vi "DAQ_ReadMeasurements.vi"(0 "task/channels in":refnum<k21>, 7 "error in":errorcluster) -> (20 "task out":refnum<k21>, 21 "Measurements":T1, 22 "Raw Temperature Voltage (V)":dbl, 23 "Raw Current Voltage (V)":dbl, 24 "Raw Torque Voltage (V)":dbl, 25 "Raw Vibration Voltage (V)":dbl, 26 "Raw RPM Voltage (V)":dbl, 27 "error out":errorcluster)   [LabVIEW 2026]
uses:
  MotorMeasurements.ctl
  <vilib>/DAQmx/read.llb/DAQmx Read (Analog 1D DBL NChan 1Samp).vi
  <vilib>/DAQmx/miscellaneous.llb/DAQmx Fill In Error Info.vi
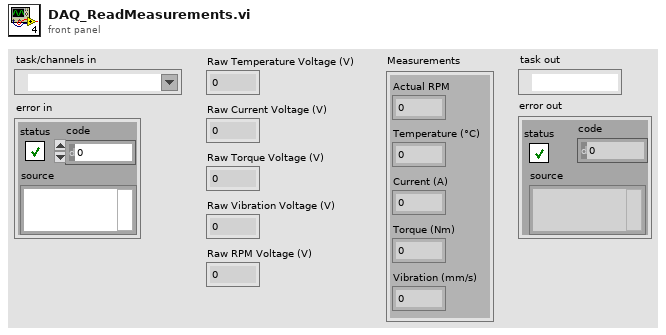
[diagram p1: front panel]
types:
  T1 = typedef "MotorMeasurements.ctl" = cluster{"Temperature (°C)":dbl, "Current (A)":dbl, "Torque (Nm)":dbl, "Vibration (mm/s)":dbl, "Actual RPM":dbl}
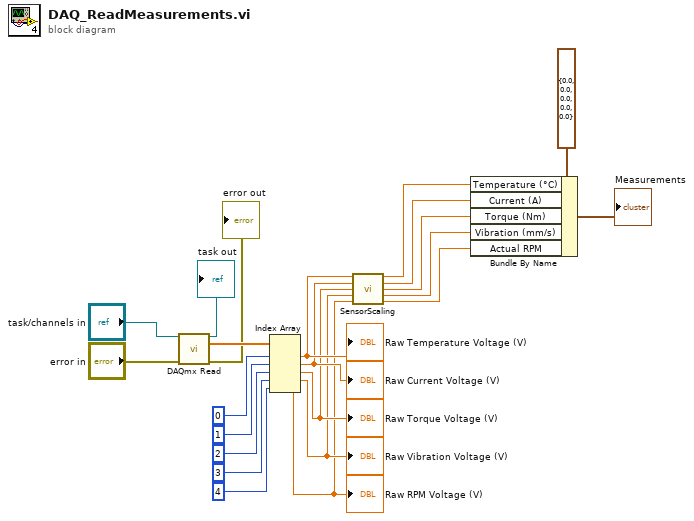
[diagram p0: block diagram]
diagram:
  n1 = call-poly <vilib>:"DAQmx Read.vi"("task/channels in"="task/channels in", "error in"="error in") -> ("task out"=→"task out":refnum<k21>, "data"=w16:dbl[], "error out"=→"error out":errorcluster)  [unwired: 11 in]
  n2 = Index Array(array=w16, index #1=0 ("index"), index #2=1 ("index"), index #3=2 ("index"), index #4=3 ("index"), index #5=4 ("index")) -> (element #1=w15:dbl, element #2=w14:dbl, element #3=w4:dbl, element #4=w3:dbl, element #5=w2:dbl)
  "Raw Temperature Voltage (V)" <- w15
  "Raw Current Voltage (V)" <- w14
  "Raw Torque Voltage (V)" <- w4
  "Raw Vibration Voltage (V)" <- w3
  "Raw RPM Voltage (V)" <- w2
  n3 = call "SensorScaling.vi"("Temperature Voltage (V)"=w15, "Current Voltage (V)"=w14, "Torque Voltage (V)"=w4, "Vibration Voltage (V)"=w3, "RPM Voltage (V)"=w2) -> ("Temperature (°C)"=w9:dbl, "Current (A)"=w8:dbl, "Torque (Nm)"=w6:dbl, "Vibration (mm/s)"=w5:dbl, "Actual RPM"=w1:dbl)  [unwired: 6 in]
  n4 = Bundle By Name(cluster=T1 {"Temperature (°C)"=0.0, "Current (A)"=0.0, "Torque (Nm)"=0.0, "Vibration (mm/s)"=0.0, "Actual RPM"=0.0} ("Measurements"), "Temperature (°C)"=w9, "Current (A)"=w8, "Torque (Nm)"=w6, "Vibration (mm/s)"=w5, "Actual RPM"=w1) -> (→"Measurements":T1)
